vi "Hybrid PS Set Control.vi"(0 "Value":variant, 1 "Change it":bool, 2 "Control Name":string="Setpoint [kA]", 3 "VI Refnum":refnum<vi>) -> ()   [LabVIEW 2019]
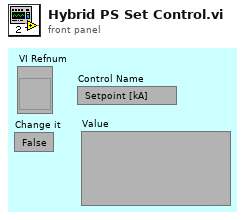
[diagram p1: front panel]
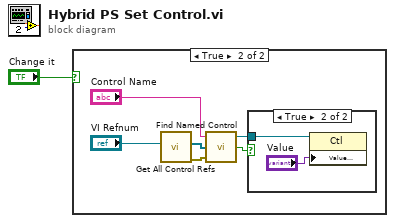
[diagram p0: block diagram]
diagram:
  n1 = case shown="True" "Change it" {
    frame False {
    }
    frame True {
      n2 = call "Get All Control Refs.vi"("vi reference"="VI Refnum") -> ("All Controls"=w3:refnum<vi>[], "error out"=w2:errorcluster)  [unwired: 5 in, 1 out]
      n3 = call "Find Named Control.vi"("error in"=w2, "All Controls"=w3, "Control Name"="Control Name") -> ("Found"=w6:bool, "Ctl Refnum"=w7:refnum<vi>)  [unwired: 1 out]
      n4 = case shown="True" w6 {
        tunnel: w7 -> [_ w9]
        frame False {
        }
        frame True {
          n5 = property class="Ctl"(reference=w9, "Value (Signaling)"="Value") -> ()  [unwired: 1 in, 2 out]
        }
      }
    }
  }
